vi "Configure Trigger.vi"(0 "VISA resource name":refnum<visa-resource-name>, 1 "Trigger Type (0:Untriggered)":u16(ring) items=["Untriggered", "Software Triggered", "Hardware Triggered"], 5 "Trigger Start Edge (0: Rising)":u16(ring) items=["Rising", "Falling"], 7 "Trigger Stop Edge (0: Rising)":u16(ring) items=["Rising", "Falling"], 9 "Trigger Stop Condition (1:Edge Triggering)":u16(ring)=1 items=["Number of Acquisitions", "Edge Triggering"], 11 "error in (no error)":errorcluster, 12 "Number of Acquisitions (100)":i32=100, 13 "Enable Continuous Trigger (Disabled)":bool) -> (4 "VISA resource name out":refnum<visa-resource-name>, 15 "error out":errorcluster)   [LabVIEW 2015, in "Micron Optics sm130.lvlib"]
doc: "Configures the trigger settings such as trigger type, start and stop edge, stop conditions, number of acquisitions and enable continuous trigger."
uses:
  Micron Optics sm130.lvlib
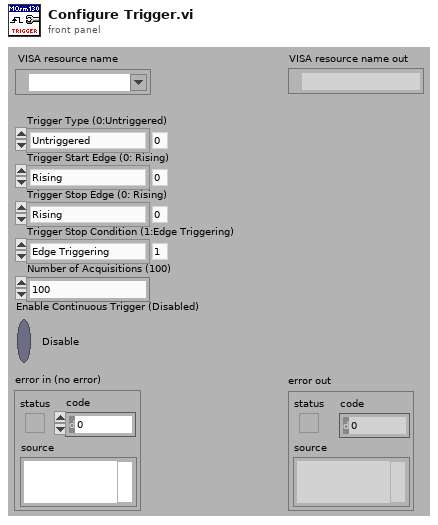
[diagram p1: front panel]
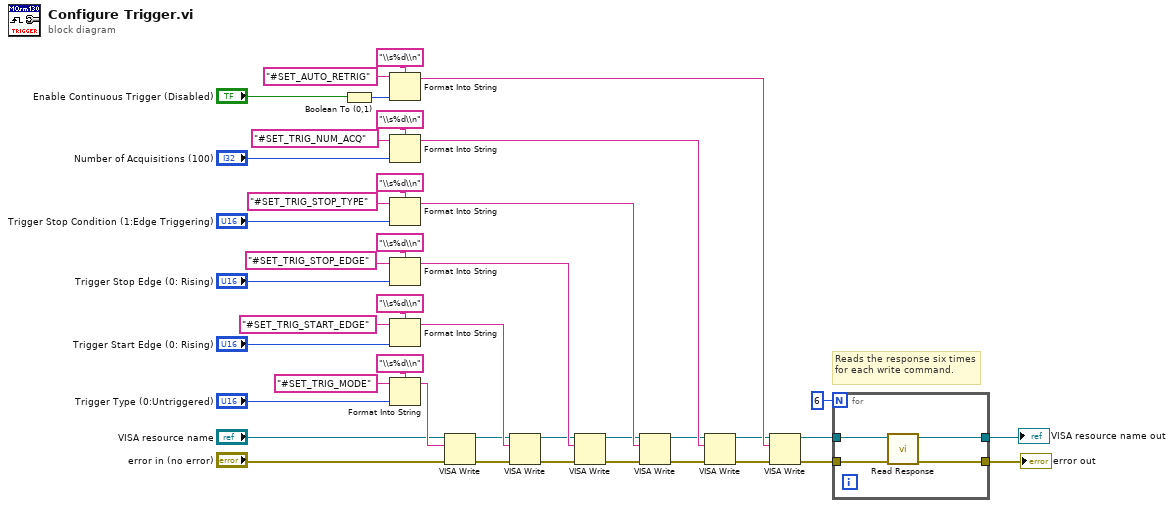
[diagram p0: block diagram]
diagram:
  # "Reads the response six times for each write command."
  n1 = Boolean To (0,1)(Boolean="Enable Continuous Trigger (Disabled)") -> (0, 1=w23:i16)
  n2 = Format Into String(format string="\\s%d\\n", initial string="#SET_AUTO_RETRIG", w23) -> (resulting string=w18:string)  [unwired: 1 in, 1 out]
  n3 = Format Into String(format string="\\s%d\\n", initial string="#SET_TRIG_NUM_ACQ", "Number of Acquisitions (100)") -> (resulting string=w19:string)  [unwired: 1 in, 1 out]
  n4 = Format Into String(format string="\\s%d\\n", initial string="#SET_TRIG_STOP_TYPE", "Trigger Stop Condition (1:Edge Triggering)") -> (resulting string=w20:string)  [unwired: 1 in, 1 out]
  n5 = Format Into String(format string="\\s%d\\n", initial string="#SET_TRIG_STOP_EDGE", "Trigger Stop Edge (0: Rising)") -> (resulting string=w21:string)  [unwired: 1 in, 1 out]
  n6 = Format Into String(format string="\\s%d\\n", initial string="#SET_TRIG_START_EDGE", "Trigger Start Edge (0: Rising)") -> (resulting string=w22:string)  [unwired: 1 in, 1 out]
  n7 = Format Into String(format string="\\s%d\\n", initial string="#SET_TRIG_MODE", "Trigger Type (0:Untriggered)") -> (resulting string=w39:string)  [unwired: 1 in, 1 out]
  n8 = VISA Write(VISA resource name="VISA resource name", write buffer=w39, error in (no error)="error in (no error)") -> (VISA resource name out=w6:refnum<visa-resource-name>, error out=w5:errorcluster)  [unwired: 1 out]
  n9 = VISA Write(VISA resource name=w6, write buffer=w22, error in (no error)=w5) -> (VISA resource name out=w8:refnum<visa-resource-name>, error out=w7:errorcluster)  [unwired: 1 out]
  n10 = VISA Write(VISA resource name=w8, write buffer=w21, error in (no error)=w7) -> (VISA resource name out=w9:refnum<visa-resource-name>, error out=w10:errorcluster)  [unwired: 1 out]
  n11 = VISA Write(VISA resource name=w9, write buffer=w20, error in (no error)=w10) -> (VISA resource name out=w12:refnum<visa-resource-name>, error out=w11:errorcluster)  [unwired: 1 out]
  n12 = VISA Write(VISA resource name=w12, write buffer=w19, error in (no error)=w11) -> (VISA resource name out=w14:refnum<visa-resource-name>, error out=w13:errorcluster)  [unwired: 1 out]
  n13 = VISA Write(VISA resource name=w14, write buffer=w18, error in (no error)=w13) -> (VISA resource name out=w16:refnum<visa-resource-name>, error out=w15:errorcluster)  [unwired: 1 out]
  n14 = for {
    N: 6 -> [_]
    tunnel: w16 -> [w46]
    tunnel: w15 -> [w45]
    tunnel: [w44] -> w2
    tunnel: [w43] -> w1
    n15 = call "Read Response.vi"("error in (no error)"=w45, "VISA resource name"=w46) -> ("error out"=w43:errorcluster, "VISA resource name out"=w44:refnum<visa-resource-name>)  [unwired: 7 in, 1 out]
  }
  "VISA resource name out" <- w2
  "error out" <- w1
